vi "varXNode_CheckForRTFIFOMutationAndIssueWarning.vi"(9 "Replies in":string[](array[string]), 11 "State":T1) -> (1 "Replies out":string[](array[string]))   [LabVIEW 2020, in "varXNode.xnode"]
uses:
  <vilib>/variable/varXNode.llb/varXNode.xnode
  <vilib>/variable/varXNode.llb/varXNode_old_8_1_0_0.ctl
  <vilib>/variable/Type Descriptor.ctl
  <vilib>/XNodeSupport/NI_XNodeSupport.lvlib
  <vilib>/variable/NI_Variable.lvlib
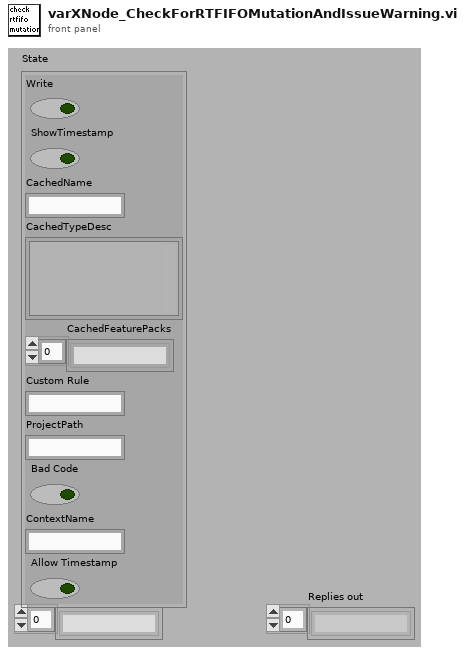
[diagram p1: front panel]
types:
  T1 = typedef "varXNode.xnode/varXNode_old_8_1_0_0.ctl" = cluster{"Write":bool, "ShowTimestamp":bool, "CachedName":string, "CachedTypeDesc":T2, "CachedFeaturePacks":string[], "Custom Rule":string, "ProjectPath":string, "Bad Code":bool, "ContextName":string, "Allow Timestamp":bool}
  T2 = typedef "NI_Variable.lvlib/Type Descriptor.ctl" = cluster{"Variant":variant}
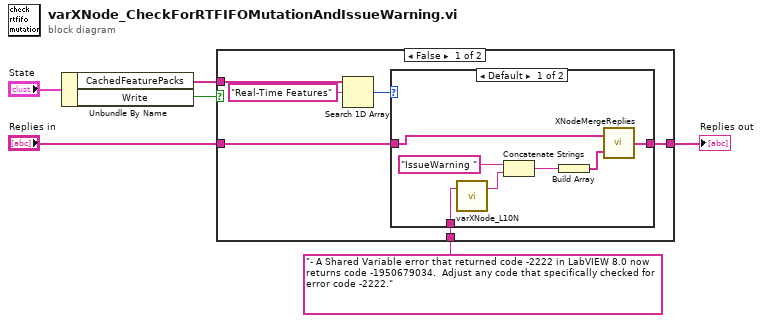
[diagram p0: block diagram]
diagram:
  n1 = Unbundle By Name("State") -> ("CachedFeaturePacks"=w3:string[], "Write"=w5:bool)
  n2 = case shown="False" w5 {
    tunnel: "Replies in" -> [w9 w21]
    tunnel: [w8 w21] -> w2
    tunnel: w3 -> [w12 _]
    tunnel: "- A Shared Variable error that returned code -2222 in LabVIEW 8.0 now returns code -1950679034.  Adjust any code that specifically checked for error code -2222." ("String") -> [w7 _]
    frame False {
      n3 = Search 1D Array(1D array=w12, element="Real-Time Features") -> (index of element=w10:i32)  [unwired: 1 in]
      n4 = case shown="Default" w10 {
        tunnel: w9 -> [w19 w20]
        tunnel: [w18 w20] -> w8
        tunnel: w7 -> [w13 _]
        frame Default {
          n5 = call <vilib>:"varXNode_L10N.vi"("String In"=w13) -> ("String Out"=w16:string)  [unwired: 2 in]
          n6 = Concatenate Strings("IssueWarning " ("String"), w16) -> (w15:string)
          n7 = Build Array(w15) -> (w14:string[])
          n8 = call <vilib>:"XNodeMergeReplies.vi"("New Replies"=w14, "Old Replies"=w19) -> ("Merged Replies"=w18:string[])
        }
        frame -1 {
        }
      }
    }
    frame True {
    }
  }
  "Replies out" <- w2
